vi "DiscoveryServiceTest.vi"() -> ()   [LabVIEW 2017]
uses:
  vsws_api/vsws.lvlib
panel:
  out "Discovered":string[](array[string])
  in  "error in (no error)":errorcluster
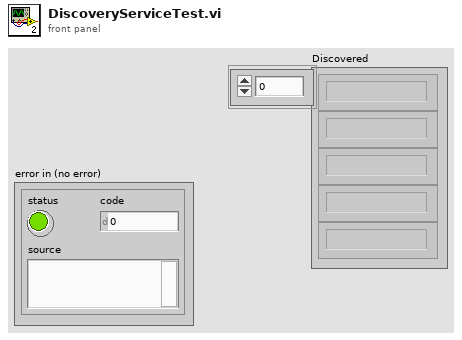
[diagram p1: front panel]
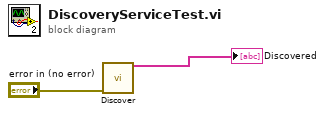
[diagram p0: block diagram]
diagram:
  n1 = call "Discover.vi"("error in (no error)"="error in (no error)") -> ("Discovered"=→"Discovered":string[])  [unwired: 13 in, 1 out]
